vi "Display Folder.vi"(8 "error in (no error)":errorcluster, 9 "Parent Tag":string, 10 "Folder in":path, 11 "TreeControl in":refnum<vi>) -> (0 "error out":errorcluster, 1 "Has Child":bool, 3 "TreeControl out":refnum<vi>)   [LabVIEW 2015, in "Editor.lvclass"]
uses:
  Editor.lvclass
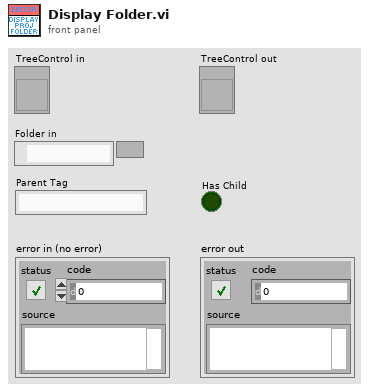
[diagram p1: front panel]
types:
  T1 = typedef "imagedata.ctl" = cluster{"image type":i32, "image depth":i32, "image":u8[], "mask":u8[], "colors":u32[], "Rectangle":cluster{"left":i16, "top":i16, "right":i16, "bottom":i16}}
  T2 = enum16{"EMPTY", "FOLDER", "VI", "CONTROL", "EXE", "IMG", "TXT"}
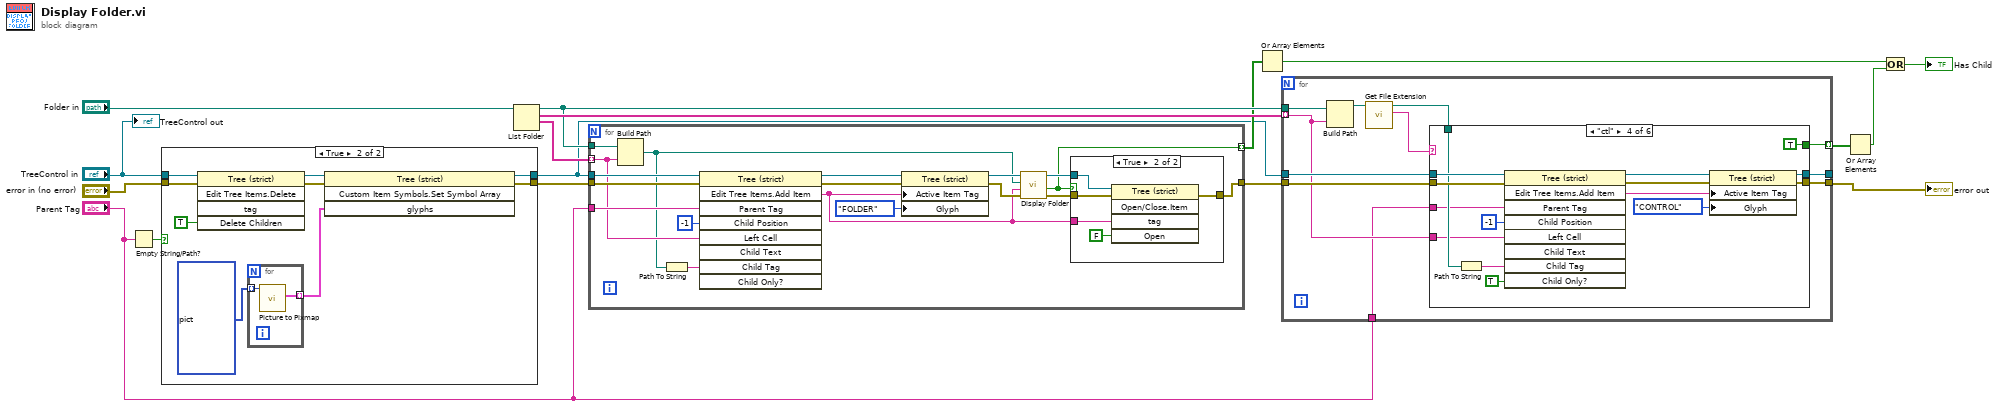
[diagram p0: block diagram]
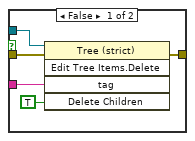
[diagram p3: hidden frame]
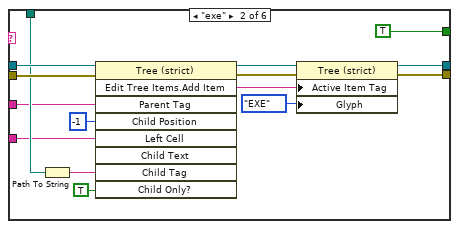
[diagram p5: hidden frame]
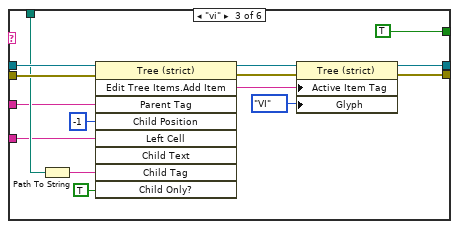
[diagram p6: hidden frame]
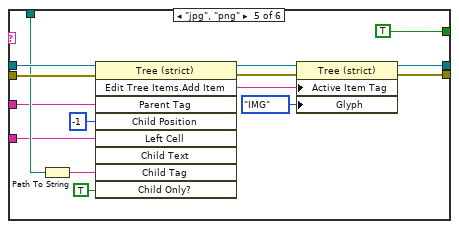
[diagram p7: hidden frame]
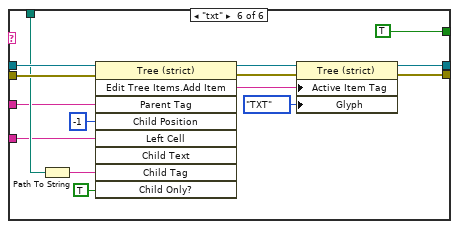
[diagram p8: hidden frame]
diagram:
  n1 = Empty String/Path?(string/path="Parent Tag") -> (empty?=w6:bool)
  n2 = case shown="True" w6 {
    tunnel: "TreeControl in" -> [w19 w27]
    tunnel: "error in (no error)" -> [w18 w26]
    tunnel: [w19 w24] -> w3
    tunnel: [w18 w22] -> w2
    frame False {
    }
    frame True {
      n3 = invoke class="Tree (strict)" method="Edit Tree Items.Delete"(reference=w27, error in=w26, "Delete Children"=TRUE ("Delete Children?")) -> (reference out=w25:refnum<vi>, error out=w23:errorcluster)  [unwired: 2 in, 3 out]
      n4 = for {
        tunnel: picture[] [bytes[0], bytes[830], bytes[830], bytes[552], bytes[702], bytes[830], bytes[830]] -> [w30] mode=indexing
        tunnel: [w29] -> w20 mode=indexing
        n5 = call <vilib>:"Picture to Pixmap.vi"("picture"=w30) -> ("image data"=w29:T1)  [unwired: 9 in, 1 out]
      }
      n6 = invoke class="Tree (strict)" method="Custom Item Symbols.Set Symbol Array"(reference=w25, error in=w23, "glyphs"=w20) -> (reference out=w24:refnum<vi>, error out=w22:errorcluster)  [unwired: 1 in, 2 out]
    }
  }
  n7 = List Folder(path="Folder in") -> (path out=w12:path, filenames=w14:string[], folder names=w15:string[])  [unwired: 3 in, 1 out]
  n8 = for {
    tunnel: w15 -> [w43] mode=indexing
    tunnel: w3 -> [w48]
    tunnel: "Parent Tag" -> [w47]
    tunnel: w2 -> [w46]
    tunnel: [w33] -> w16
    tunnel: w12 -> [w41]
    tunnel: [w32] -> w11 mode=indexing
    n9 = Build Path(base path=w41, name or relative path=w43) -> (appended path=w38:path)
    n10 = Path To String(path=w38) -> (string=w42:string)
    n11 = invoke class="Tree (strict)" method="Edit Tree Items.Add Item"(reference=w48, error in=w46, "Parent Tag"=w47, "Child Position"=-1, "Left Cell"=w43, "Child Tag"=w42) -> (reference out=w45:refnum<vi>, error out=w44:errorcluster, "Edit Tree Items:Add Item"=w34:string)  [unwired: 3 in, 6 out]
    n12 = property class="Tree (strict)"(reference=w45, error in=w44, "Active Item Tag"=w34, "Glyph"=T2."FOLDER") -> (reference out=w39:refnum<vi>, error out=w40:errorcluster)
    n13 = call "Display Folder.vi"("error in (no error)"=w40, "Parent Tag"=w34, "Folder in"=w38, "TreeControl in"=w39) -> ("error out"=w35:errorcluster, "Has Child"=w32:bool, "TreeControl out"=w36:refnum<vi>)  [unwired: 5 in]
    n14 = case shown="True" w32 {
      tunnel: w36 -> [w53 w58]
      tunnel: w35 -> [w52 w57]
      tunnel: w34 -> [w51 w56]
      tunnel: [w50 w55] -> w33
      frame False {
        n15 = invoke class="Tree (strict)" method="Edit Tree Items.Delete"(reference=w53, error in=w52, "tag"=w51, "Delete Children"=TRUE ("Delete Children?")) -> (error out=w50:errorcluster)  [unwired: 1 in, 4 out]
      }
      frame True {
        n16 = invoke class="Tree (strict)" method="Open/Close.Item"(reference=w58, error in=w57, "tag"=w56, "Open"=FALSE ("Delete Children?")) -> (error out=w55:errorcluster)  [unwired: 1 in, 4 out]
      }
    }
  }
  n17 = Or Array Elements(Boolean array=w11) -> (logical OR=w8:bool)
  n18 = for {
    tunnel: w14 -> [w65] mode=indexing
    tunnel: w3 -> [w69]
    tunnel: w16 -> [w68]
    tunnel: w12 -> [w67]
    tunnel: [w64] -> _
    tunnel: [w63] -> w13
    tunnel: "Parent Tag" -> [w60]
    tunnel: [w59] -> w10 mode=indexing
    n19 = Build Path(base path=w67, name or relative path=w65) -> (appended path=w66:path)
    n20 = call <vilib>:"Get File Extension.vi"("file"=w66) -> ("lowercase file extension"=w62:string, "dup file"=w61:path)  [unwired: 6 in, 3 out]
    n21 = case shown="\"ctl\"" w62 {
      tunnel: w69 -> [w71 w86 w101 w116 w131 w146]
      tunnel: w68 -> [w70 w85 w100 w115 w130 w145]
      tunnel: w65 -> [_ w75 w90 w105 w120 w135]
      tunnel: w61 -> [_ w81 w96 w111 w126 w141]
      tunnel: [w71 w80 w95 w110 w125 w140] -> w64
      tunnel: [w70 w79 w94 w109 w124 w139] -> w63
      tunnel: [_ TRUE TRUE TRUE TRUE TRUE] -> w59
      tunnel: w60 -> [_ w74 w89 w104 w119 w134]
      frame Default {
      }
      frame "exe" {
        n22 = Path To String(path=w81) -> (string=w76:string)
        n23 = invoke class="Tree (strict)" method="Edit Tree Items.Add Item"(reference=w86, error in=w85, "Parent Tag"=w74, "Child Position"=-1, "Left Cell"=w75, "Child Tag"=w76, "Child Only?"=TRUE) -> (reference out=w84:refnum<vi>, error out=w83:errorcluster, "Edit Tree Items:Add Item"=w82:string)  [unwired: 2 in, 6 out]
        n24 = property class="Tree (strict)"(reference=w84, error in=w83, "Active Item Tag"=w82, "Glyph"=T2."EXE") -> (reference out=w80:refnum<vi>, error out=w79:errorcluster)
      }
      frame "vi" {
        n25 = Path To String(path=w96) -> (string=w91:string)
        n26 = invoke class="Tree (strict)" method="Edit Tree Items.Add Item"(reference=w101, error in=w100, "Parent Tag"=w89, "Child Position"=-1, "Left Cell"=w90, "Child Tag"=w91, "Child Only?"=TRUE) -> (reference out=w99:refnum<vi>, error out=w98:errorcluster, "Edit Tree Items:Add Item"=w97:string)  [unwired: 2 in, 6 out]
        n27 = property class="Tree (strict)"(reference=w99, error in=w98, "Active Item Tag"=w97, "Glyph"=T2."VI") -> (reference out=w95:refnum<vi>, error out=w94:errorcluster)
      }
      frame "ctl" {
        n28 = Path To String(path=w111) -> (string=w106:string)
        n29 = invoke class="Tree (strict)" method="Edit Tree Items.Add Item"(reference=w116, error in=w115, "Parent Tag"=w104, "Child Position"=-1, "Left Cell"=w105, "Child Tag"=w106, "Child Only?"=TRUE) -> (reference out=w114:refnum<vi>, error out=w113:errorcluster, "Edit Tree Items:Add Item"=w112:string)  [unwired: 2 in, 6 out]
        n30 = property class="Tree (strict)"(reference=w114, error in=w113, "Active Item Tag"=w112, "Glyph"=T2."CONTROL") -> (reference out=w110:refnum<vi>, error out=w109:errorcluster)
      }
      frame "jpg", "png" {
        n31 = Path To String(path=w126) -> (string=w121:string)
        n32 = invoke class="Tree (strict)" method="Edit Tree Items.Add Item"(reference=w131, error in=w130, "Parent Tag"=w119, "Child Position"=-1, "Left Cell"=w120, "Child Tag"=w121, "Child Only?"=TRUE) -> (reference out=w129:refnum<vi>, error out=w128:errorcluster, "Edit Tree Items:Add Item"=w127:string)  [unwired: 2 in, 6 out]
        n33 = property class="Tree (strict)"(reference=w129, error in=w128, "Active Item Tag"=w127, "Glyph"=T2."IMG") -> (reference out=w125:refnum<vi>, error out=w124:errorcluster)
      }
      frame "txt" {
        n34 = Path To String(path=w141) -> (string=w136:string)
        n35 = invoke class="Tree (strict)" method="Edit Tree Items.Add Item"(reference=w146, error in=w145, "Parent Tag"=w134, "Child Position"=-1, "Left Cell"=w135, "Child Tag"=w136, "Child Only?"=TRUE) -> (reference out=w144:refnum<vi>, error out=w143:errorcluster, "Edit Tree Items:Add Item"=w142:string)  [unwired: 2 in, 6 out]
        n36 = property class="Tree (strict)"(reference=w144, error in=w143, "Active Item Tag"=w142, "Glyph"=T2."TXT") -> (reference out=w140:refnum<vi>, error out=w139:errorcluster)
      }
    }
  }
  "error out" <- w13
  n37 = Or Array Elements(Boolean array=w10) -> (logical OR=w9:bool)
  n38 = Or(x=w8, y=w9) -> (x .or. y?=→"Has Child":bool)
  "TreeControl out" <- "TreeControl in"
